vi "GetOffs.vi"(11 "RefIn":refnum<file>) -> (0 "HeightOff":u32, 1 "IntenOff":u32, 2 "LOoff":u32, 3 "OpticalOff":u32, 4 "RefOut":refnum<file>)   [LabVIEW 2014]
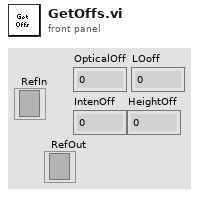
[diagram p1: front panel]
types:
  T1 = enum16{"big-endian, network order", "native, host order", "little-endian"}
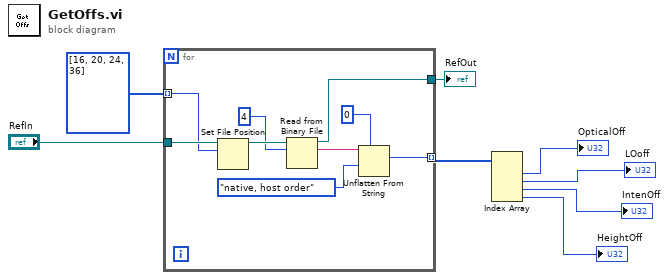
[diagram p0: block diagram]
diagram:
  n1 = for {
    tunnel: "RefIn" -> [w17]
    tunnel: i32[] [16, 20, 24, 36] -> [w14] mode=indexing
    tunnel: [w11] -> w7 mode=indexing
    tunnel: [w9] -> w1
    n2 = Set File Position(offset (in bytes) (0)=w14, refnum=w17) -> (refnum out=w16:refnum<file>)  [unwired: 2 in, 1 out]
    n3 = Read from Binary File(10:4 ("count (1)"), 11:w16) -> (2:w13:string, 3:w9:refnum<file>)  [unwired: 4 in, 2 out]
    n4 = Unflatten From String(type=u32 0, binary string=w13, byte order (0:big-endian, network order)=T1."native, host order") -> (value=w11:u32)  [unwired: 2 in, 2 out]
  }
  "RefOut" <- w1
  n5 = Index Array(array=w7) -> (element #1=→"OpticalOff":u32, element #2=→"LOoff":u32, element #3=→"IntenOff":u32, element #4=→"HeightOff":u32)  [unwired: 4 in]
